vi "Binary Search on One Hot Encoded Number (U32).vi"(7 "One Hot Encoded Number":u32 format="%032b") -> (8 "Binary Number":u8)   [LabVIEW 2011]
doc: "This VI gives the index the index of first one from LSB. It assumes that the number is one hot encoded.\nInother words it converts one hot encoded number to Binary Number"
panel:
  out "a[3]":bool
  out "a[4]":bool
  out "Binary Array":bool[](array[boolean])
  out "a[0]":bool
  out "a[1]":bool
  out "a[2]":bool
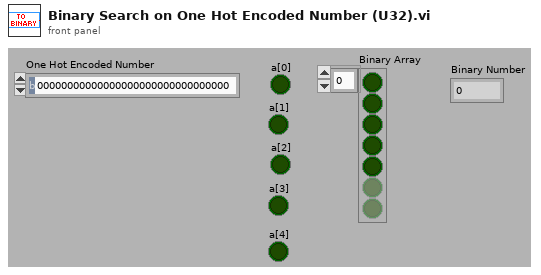
[diagram p1: front panel]
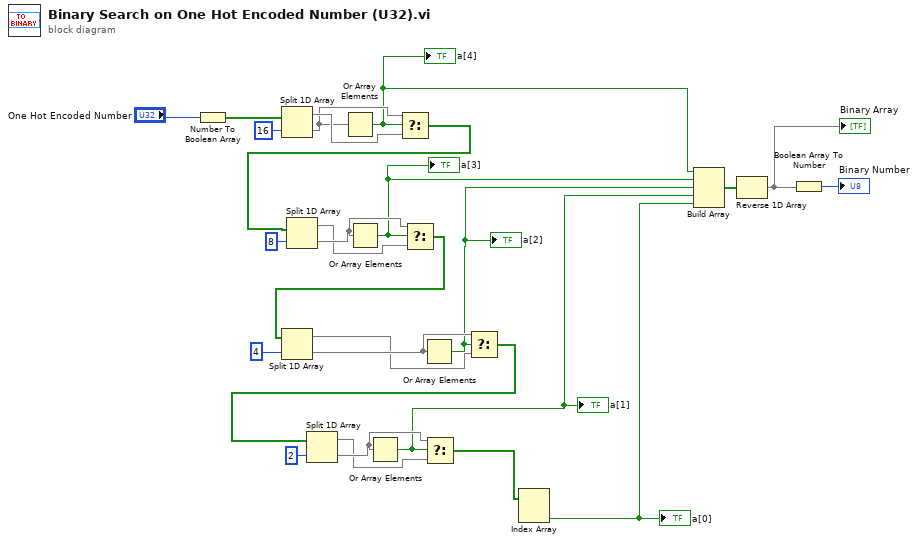
[diagram p0: block diagram]
diagram:
  n1 = Number To Boolean Array(number="One Hot Encoded Number") -> (Boolean array=w9:bool[])
  n2 = Split 1D Array(array=w9, index=16) -> (first subarray=w12:bool[], second subarray=w11:bool[])
  n3 = Or Array Elements(Boolean array=w11) -> (logical OR=w3:bool)
  "a[4]" <- w3
  n4 = Select(t=w11, s=w3, f=w12) -> (s? t:f=w5:bool[])
  n5 = Split 1D Array(array=w5, index=8) -> (first subarray=w6:bool[], second subarray=w7:bool[])
  n6 = Or Array Elements(Boolean array=w7) -> (logical OR=w1:bool)
  "a[3]" <- w1
  n7 = Select(t=w7, s=w1, f=w6) -> (s? t:f=w4:bool[])
  n8 = Split 1D Array(array=w4, index=4) -> (first subarray=w24:bool[], second subarray=w25:bool[])
  n9 = Or Array Elements(Boolean array=w25) -> (logical OR=w2:bool)
  "a[2]" <- w2
  n10 = Select(t=w25, s=w2, f=w24) -> (s? t:f=w23:bool[])
  n11 = Split 1D Array(array=w23, index=2) -> (first subarray=w20:bool[], second subarray=w21:bool[])
  n12 = Or Array Elements(Boolean array=w21) -> (logical OR=w19:bool)
  "a[1]" <- w19
  n13 = Select(t=w21, s=w19, f=w20) -> (s? t:f=w15:bool[])
  n14 = Index Array(array=w15) -> (element #2=w14:bool)  [unwired: 2 in, 1 out]
  "a[0]" <- w14
  n15 = Build Array(w3, w1, w2, w19, w14) -> (w18:bool[])
  n16 = Reverse 1D Array(array=w18) -> (reversed array=w16:bool[])
  "Binary Array" <- w16
  n17 = Boolean Array To Number(Boolean array=w16) -> (number=→"Binary Number":u8)
